vi "FTW-Menu-TagDecode.vi"(0 "Menu Item Tag":string) -> (2 "Class":string, 3 "Command":string, 4 "Payload":string)   [LabVIEW 2013]
panel:
  # "Inputs"
  # "Outputs"
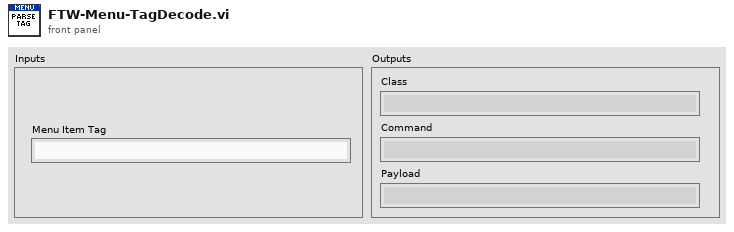
[diagram p1: front panel]
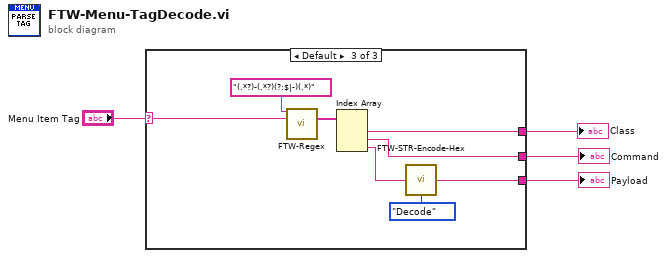
[diagram p0: block diagram]
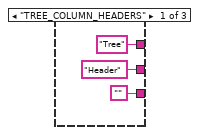
[diagram p2: hidden frame]
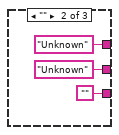
[diagram p3: hidden frame]
diagram:
  n1 = case shown="Default" "Menu Item Tag" {
    selector: "Menu Item Tag" -> [_ _ w11]
    tunnel: ["Tree" ("Submatch") "Unknown" ("Submatch") w16] -> w4
    tunnel: ["Header" ("Submatch") "Unknown" ("Submatch") w15] -> w3
    tunnel: ["" "" w13] -> w2
    frame "TREE_COLUMN_HEADERS" {
    }
    frame "" {
    }
    frame Default {
      n2 = call "FTW-Regex.vi"("Regular Expression"="(.*?)-(.*?)(?:$|-)(.*)" ("regular expression"), "Input String"=w11) -> ("Submatches"=w17:string[])  [unwired: 9 in, 4 out]
      n3 = Index Array(array=w17) -> (element #1=w16:string, element #2=w15:string, element #3=w14:string)  [unwired: 3 in]
      n4 = call "FTW-STR-Encode-Hex.vi"("Input"=w14, "Direction"=enum16{"Encode", "Decode"}."Decode") -> ("Output"=w13:string)
    }
  }
  "Payload" <- w2
  "Command" <- w3
  "Class" <- w4
